vi "FlashA-B.vi"(8 "error in":errorcluster caption="错误输入", 11 "Setup":T1) -> (0 "error out":errorcluster caption="错误输出")   [LabVIEW 2013]
uses:
  SetupCtl.ctl
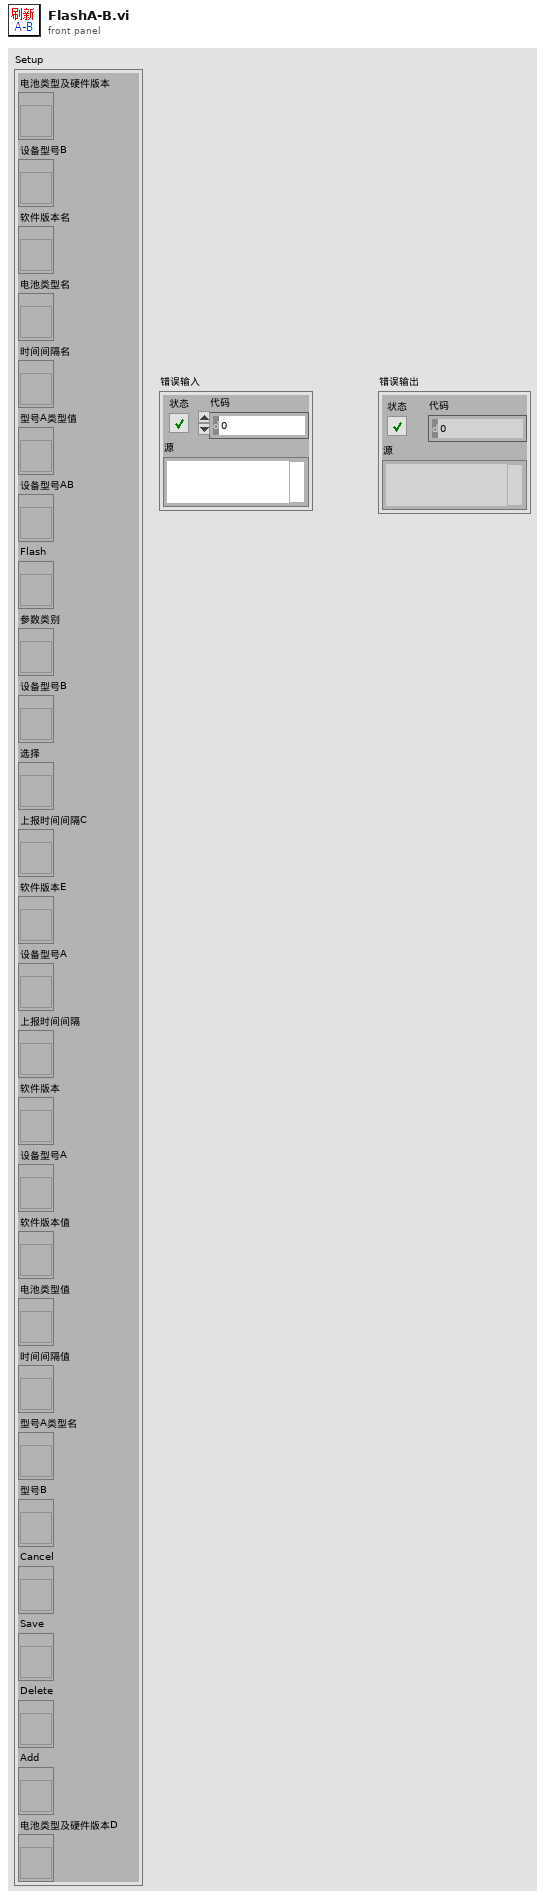
[diagram p1: front panel]
types:
  T1 = typedef "SetupCtl.ctl" = cluster{"电池类型及硬件版本":refnum<vi>, "设备型号B":refnum<vi>, "软件版本名":refnum<vi>, "电池类型名":refnum<vi>, "时间间隔名":refnum<vi>, "型号A类型值":refnum<vi>, "设备型号AB":refnum<vi>, "Flash":refnum<vi>, "参数类别":refnum<vi>, "设备型号B":refnum<vi>, "选择":refnum<vi>, "上报时间间隔C":refnum<vi>, "软件版本E":refnum<vi>, "设备型号A":refnum<vi>, "上报时间间隔":refnum<vi>, "软件版本":refnum<vi>, "设备型号A":refnum<vi>, "软件版本值":refnum<vi>, "电池类型值":refnum<vi>, "时间间隔值":refnum<vi>, "型号A类型名":refnum<vi>, "型号B":refnum<vi>, "Cancel":refnum<vi>, "Save":refnum<vi>, "Delete":refnum<vi>, "Add":refnum<vi>, "电池类型及硬件版本D":refnum<vi>}
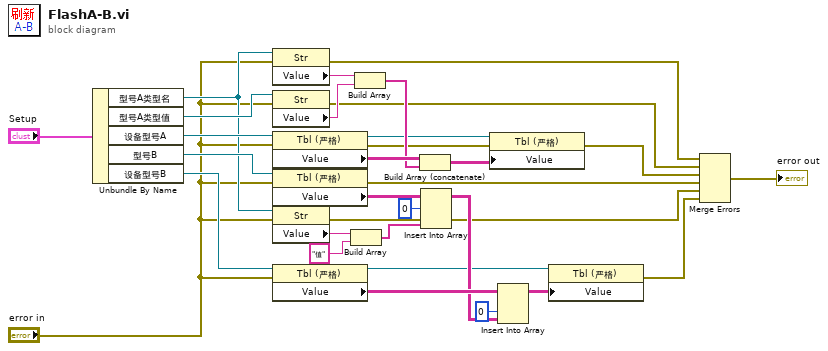
[diagram p0: block diagram]
diagram:
  n1 = Unbundle By Name("Setup") -> ("型号A类型名"=w21:refnum<vi>, "型号A类型值"=w30:refnum<vi>, "设备型号A"=w27:refnum<vi>, "型号B"=w22:refnum<vi>, "设备型号B"=w15:refnum<vi>)
  n2 = property class="Str"(reference=w21, error in="error in") -> (error out=w7:errorcluster, "Value"=w29:string)  [unwired: 1 out]
  n3 = property class="Str"(reference=w30, error in="error in") -> (error out=w6:errorcluster, "Value"=w28:string)  [unwired: 1 out]
  n4 = property class="Tbl (严格)"(reference=w27, error in="error in") -> (reference out=w24:refnum<vi>, error out=w8:errorcluster, "Value"=w26:string[][])
  n5 = property class="Tbl (严格)"(reference=w22, error in="error in") -> (error out=w4:errorcluster, "Value"=w18:string[][])  [unwired: 1 out]
  n6 = property class="Str"(reference=w21, error in="error in") -> (error out=w3:errorcluster, "Value"=w20:string)  [unwired: 1 out]
  n7 = property class="Tbl (严格)"(reference=w15, error in="error in") -> (reference out=w11:refnum<vi>, "Value"=w14:string[][])  [unwired: 1 out]
  n8 = Build Array(w20, "值") -> (w16:string[])
  n9 = Build Array(w29, w28) -> (w25:string[])
  n10 = Build Array (concatenate)(w26, w25) -> (w23:string[][])
  n11 = Insert Into Array(array=w18, index (row)=0 ("索引 (行)"), new element=w16) -> (w12:string[][])  [unwired: 1 in]
  n12 = property class="Tbl (严格)"(reference=w24, error in=w8, "Value"=w23) -> (error out=w5:errorcluster)  [unwired: 1 out]
  n13 = Insert Into Array(array=w14, index (col)=0 ("禁用的索引 (列)"), new element=w12) -> (w10:string[][])  [unwired: 1 in]
  n14 = property class="Tbl (严格)"(reference=w11, "Value"=w10) -> (error out=w2:errorcluster)  [unwired: 1 in, 1 out]
  n15 = Merge Errors(w7, w6, w5, w4, w3, w2) -> (→"error out":errorcluster)
